vi "config_timebase_OSC_new.vi"(8 "error in (no error)":errorcluster, 9 "resolution":i32=10000 caption="Record Length (10000s)", 10 "hor scale":dbl, 11 "VISA resource name":refnum<visa-resource-name>) -> (0 "error out":errorcluster, 3 "VISA resource name out":refnum<visa-resource-name>)   [LabVIEW 2011]
doc: "Configures the timebase and horizontal properties of an oscilloscope."
panel:
  in  "sample rate":ext
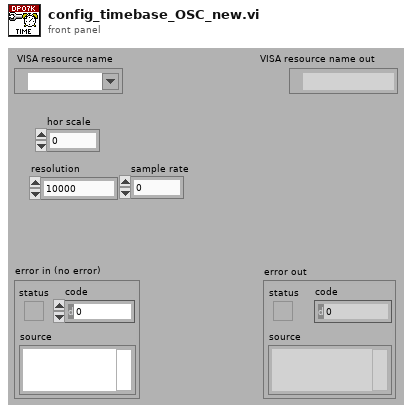
[diagram p1: front panel]
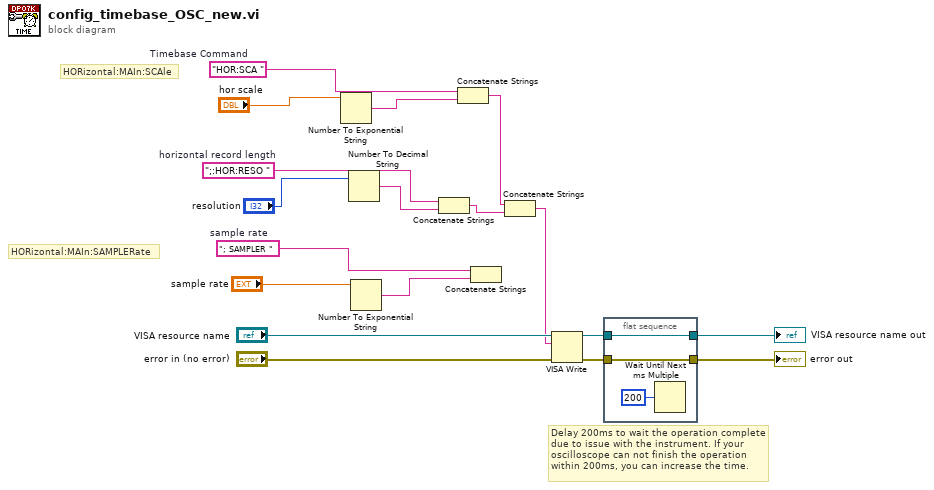
[diagram p0: block diagram]
diagram:
  w4 = "; SAMPLER "  # sample rate
  w8 = ";:HOR:RESO "  # horizontal record length
  w12 = "HOR:SCA "  # Timebase Command
  # "HORizontal:MAIn:SCAle"
  # "HORizontal:MAIn:SAMPLERate"
  # "Delay 200ms to wait the operation complete due to issue with the instrument. If your oscilloscope can not finish the operation within 200ms, you can increase the time."
  n1 = Number To Exponential String(number="hor scale") -> (E-format string=w11:string)  [unwired: 3 in]
  n2 = Number To Decimal String(number="resolution") -> (decimal integer string=w7:string)  [unwired: 1 in]
  n3 = Number To Exponential String(number="sample rate") -> (E-format string=w3:string)  [unwired: 3 in]
  n4 = Concatenate Strings(w8, w7) -> (w1:string)
  n5 = Concatenate Strings(w12, w11) -> (w6:string)
  n6 = Concatenate Strings(w4, w3) -> ()  [unwired: 1 out]
  n7 = Concatenate Strings(w6, w1) -> (w5:string)
  n8 = VISA Write(VISA resource name="VISA resource name", write buffer=w5, error in (no error)="error in (no error)") -> (VISA resource name out=w17:refnum<visa-resource-name>, error out=w16:errorcluster)  [unwired: 1 out]
  n9 = flat-sequence {
    tunnel: w17 -> [w20]
    tunnel: [w20] -> w14
    tunnel: w16 -> [w19]
    tunnel: [w19] -> w13
    frame #0 {
      n10 = Wait Until Next ms Multiple(millisecond multiple=u32 200) -> ()  [unwired: 1 out]
    }
  }
  "VISA resource name out" <- w14
  "error out" <- w13
